vi "AutoTune.vi"(7 "Input Auto Freq Array":dbl[](array[numeric]), 9 "Autotune?":bool, 10 "Input Freq":dbl) -> (2 "Output AutoTuned Freq":dbl)   [LabVIEW 2012]
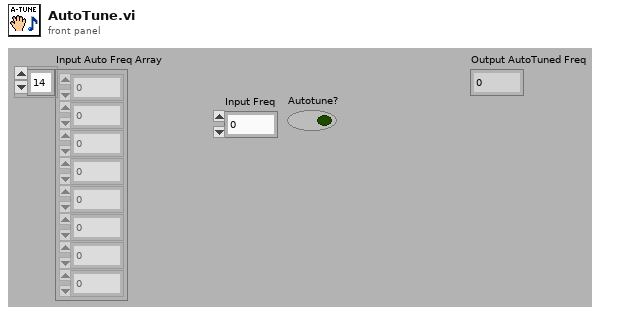
[diagram p1: front panel]
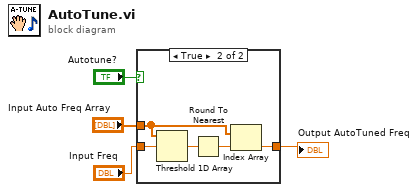
[diagram p0: block diagram]
diagram:
  n1 = case shown="True" "Autotune?" {
    tunnel: [w5 w7] -> w4
    tunnel: "Input Auto Freq Array" -> [_ w9]
    tunnel: "Input Freq" -> [w5 w10]
    frame False {
    }
    frame True {
      n2 = Threshold 1D Array(2:w10, 3:w9) -> (0:w6:dbl)  [unwired: 1 in]
      n3 = Round To Nearest(number=w6) -> (nearest integer value=w8:dbl)
      n4 = Index Array(array=w9, index=w8) -> (element=w7:dbl)
    }
  }
  "Output AutoTuned Freq" <- w4
